vi "FindLeakPeak.vi"(7 "坐标关系":T1, 9 "n 等分倍数":dbl format="%#.6g", 10 "Zi":dbl[][](array[numeric]), 11 "渗漏点":refnum<vi>) -> (1 "绘图坐标Y":dbl format="%#.6g", 2 "最大值":dbl, 3 "最大索引":u32[](array[numeric]), 4 "绘图坐标X":dbl format="%#.6g")   [LabVIEW 2014, in "cyy.lvlib" / "LeakageFenXi.lvlib"]
uses:
  LeakageFenXi.lvlib
panel:
  out "Y":dbl format="%#.6g"
  out "X":dbl format="%#.6g"
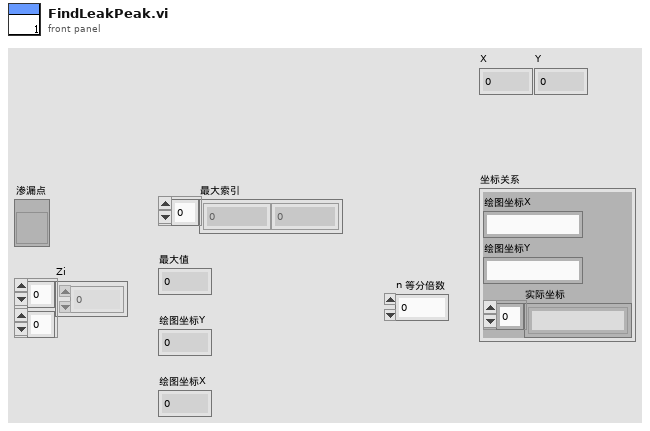
[diagram p1: front panel]
types:
  T1 = cluster{"绘图坐标X":string, "绘图坐标Y":string, "实际坐标":string[]}
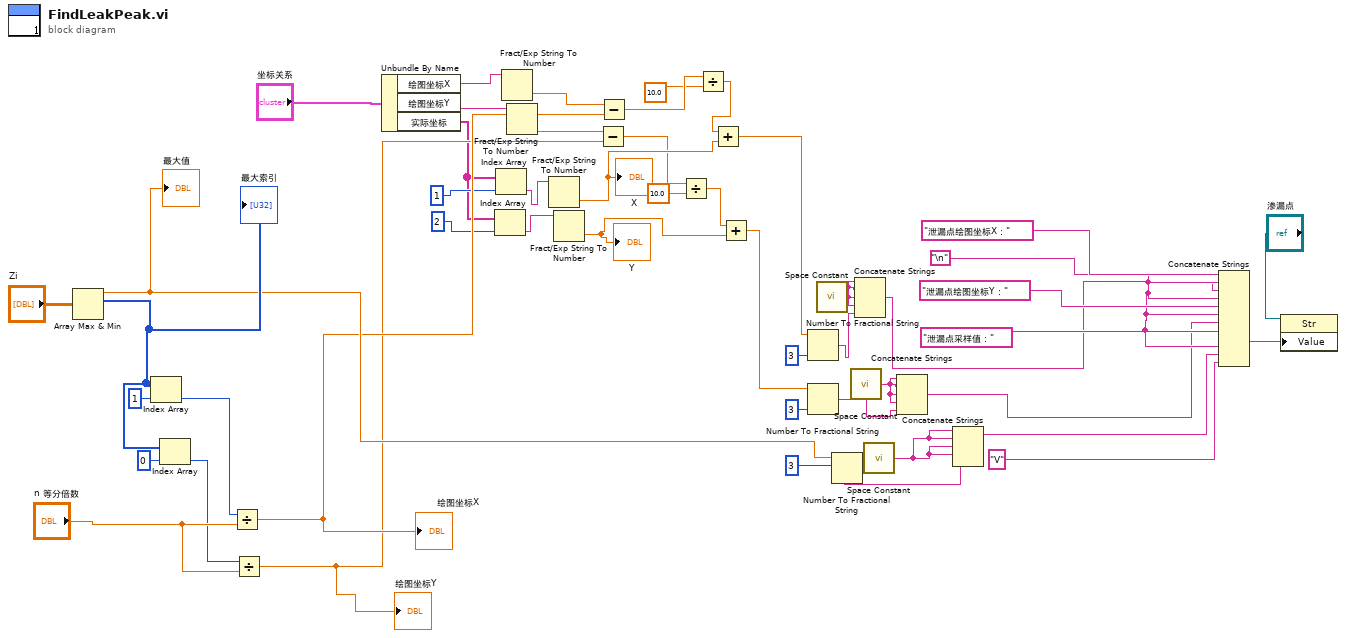
[diagram p0: block diagram]
diagram:
  w40 = "\n"
  n1 = Array Max & Min(array="Zi") -> (max value=w34:dbl, max index (indices)=w46:i32[])  [unwired: 2 out]
  "最大值" <- w34
  "最大索引" <- w46
  n2 = Index Array(array=w46, index=1 ("索引")) -> (element=w30:i32)
  n3 = Index Array(array=w46, index=0 ("索引")) -> (element=w28:i32)
  n4 = Divide(x=w30, y="n 等分倍数") -> (x/y=w18:dbl)
  "绘图坐标X" <- w18
  n5 = Divide(x=w28, y="n 等分倍数") -> (x/y=w16:dbl)
  "绘图坐标Y" <- w16
  n6 = Unbundle By Name("坐标关系") -> ("绘图坐标X"=w21:string, "绘图坐标Y"=w20:string, "实际坐标"=w13:string[])
  n7 = Index Array(array=w13, index=2) -> (element=w11:string)
  n8 = Index Array(array=w13, index=1) -> (element=w12:string)
  n9 = Fract/Exp String To Number(string=w21) -> (number=w19:dbl)  [unwired: 3 in, 1 out]
  n10 = Fract/Exp String To Number(string=w20) -> (number=w17:dbl)  [unwired: 3 in, 1 out]
  n11 = Fract/Exp String To Number(string=w12) -> (number=w10:dbl)  [unwired: 3 in, 1 out]
  "X" <- w10
  n12 = Fract/Exp String To Number(string=w11) -> (number=w9:dbl)  [unwired: 3 in, 1 out]
  "Y" <- w9
  n13 = Subtract(x=w17, y=w16) -> (x-y=w4:dbl)
  n14 = Subtract(x=w19, y=w18) -> (x-y=w6:dbl)
  n15 = Divide(x=w4, y=10.0) -> (x/y=w2:dbl)
  n16 = Divide(x=w6, y=10.0) -> (x/y=w1:dbl)
  n17 = Add(x=w1, y=w10) -> (x+y=w8:dbl)
  n18 = Add(x=w2, y=w9) -> (x+y=w7:dbl)
  n19 = Number To Fractional String(number=w8, precision (6)=i16 3 ("精度(6)")) -> (F-format string=w27:string)  [unwired: 2 in]
  n20 = Number To Fractional String(number=w7, precision (6)=i16 3 ("精度(6)")) -> (F-format string=w26:string)  [unwired: 2 in]
  n21 = call <vilib>:"Space Constant.vi"() -> ("String"=w38:string)
  n22 = Number To Fractional String(number=w34, precision (6)=i16 3 ("精度(6)")) -> (F-format string=w32:string)  [unwired: 2 in]
  n23 = call <vilib>:"Space Constant.vi"() -> ("String"=w36:string)
  n24 = Concatenate Strings(w38, w38, w38, w38, w27) -> (w37:string)
  n25 = call <vilib>:"Space Constant.vi"() -> ("String"=w33:string)
  n26 = Concatenate Strings(w36, w36, w36, w36, w26) -> (w35:string)
  n27 = Concatenate Strings(w33, w33, w33, w33, w32) -> (w31:string)
  n28 = Concatenate Strings("泄漏点绘图坐标X：", w40, w37, w40, "泄漏点绘图坐标Y：", w40, w35, w40, "泄漏点采样值：", w40, w31, "V") -> (w48:string)
  n29 = property class="Str"(reference="渗漏点", "Value"=w48) -> ()  [unwired: 1 in, 2 out]
